vi "Digitizer Measurement.vi"(4 "delay (2.0 s)":dbl[unit]=2.0 format="%_3g", 6 "filepath":path, 7 "channel names":string="1,2", 8 "error in":errorcluster, 9 "trigger":T1={"trigger level"=30.0, "trigger type"=enum."Immediate", "Trigger Source"=enum."Immediate", "Trigger Slope"=enum."Positive"} {"trigger level" format="%.2f"}, 10 "vertical":T2={"vertical coupling"=enum."DC", "probe attenuation"=1.0, "vertical range"=10.0, "vertical offset"=0.0} {"vertical offset" format="%.4f"; "vertical range" format="%.2f"; "probe attenuation" format="%.1f"}, 11 "horizontal":T3={"number of records"=1, "reference position"=1.0, "min record length"=100000, "min sample rate"=1000000.0, "enforce realtime"=TRUE, "maximum input frequency"=-1.0} {"maximum input frequency" format="%.2f"; "min sample rate" step=1000000.0 format="%.0p"; "min record length" format="%.0p"; "reference position" format="%.1f"; "number of records" step=1}) -> (0 "error out":errorcluster, 2 "waveform array":waveform(dbl)[](array[waveform])=[{"t0"=timestamp(-9593225999.296875 s since 1904-01-01), "dt"=nan, "Y"=[]}, {"t0"=timestamp(3478177624.703125 s since 1904-01-01), "dt"=1e-06, "Y"=array[100000 elements]}])   [LabVIEW 2010]
doc: "This function performs Digitizer measurements (Configure, Read, and Close)."
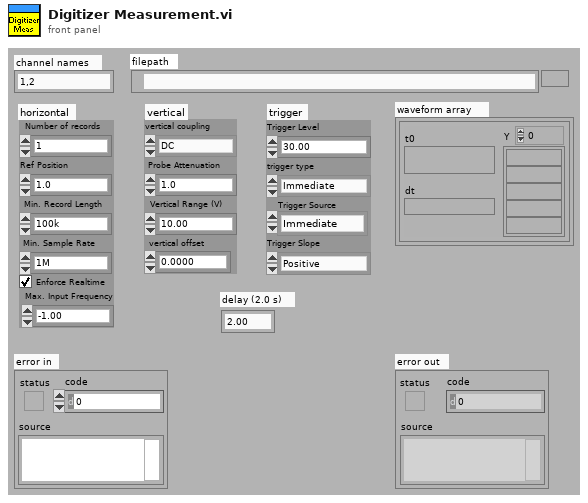
[diagram p1: front panel]
types:
  T1 = cluster{"trigger level":dbl, "trigger type":enum16{"Edge", "Digital", "Immediate"}, "Trigger Source":enum8{"Immediate", "Channel 0", "Channel 1", "Channel 2", "Channel 3", "Channel 4", "Channel 5", "Channel 6", "Channel 7", "External TRIG", "Software Trigger", "RTSI 0", "RTSI 1", "RTSI 2", "RTSI 3", "RTSI 4", "RTSI 5", "RTSI 6", "PFI 0", "PFI 1", "PFI 2", "PXI Star Trigger"}, "Trigger Slope":enum16{"Positive", "Negative"}}
  T2 = cluster{"vertical coupling":enum16{"AC", "DC", "Ground"}, "probe attenuation":dbl, "vertical range":dbl, "vertical offset":dbl}
  T3 = cluster{"number of records":i32, "reference position":dbl, "min record length":i32, "min sample rate":dbl, "enforce realtime":bool, "maximum input frequency":dbl}
  T4 = typedef "Typedef-Channel Parameters.ctl" = cluster{"Channel Name":string, "Number of Records":i32, "Reference Position":dbl, "Minimum Record Length":i32, "Minimum Sample Rate":dbl, "Maximum Input Frequency":dbl, "Enforce Realtime":bool, "Vertical Coupling":enum16{"AC", "DC", "Ground"}, "Probe Attenuation":dbl, "Vertical Range (V)":dbl, "Vertical Offset":dbl, "Trigger Level":dbl, "Trigger Type":enum16{"Edge", "Digital", "Immediate"}, "Trigger Source":enum16{"Immediate", "Channel 0", "Channel 1", "Channel 2", "Channel 3", "Channel 4", "Channel 5", "Channel 6", "Channel 7", "Extermal TRIG", "Software Trigger", "RTSI 0", "RTSI 1", "RTSI 2", "RTSI 3", "RTSI 4", "RTSI 5", "RTSI 6", "PF 0", "PF 1", "PF 2", "PXI Star Trigger"}, "Trigger Slope":enum16{"Positive", "Negative"}, "Digitizer 1 Used?":bool, "Digitizer 1 Channels":string, "Digitizer 1 Reference":refnum<k15>, "Digitizer 1 Gain Multiplier":dbl, "Digitizer 2 Used?":bool, "Digitizer 2 Channels":string, "Digitizer 2 Reference":refnum<k15>, "Session References":refnum<k20>[]}
  T5 = cluster{"relativeInitialX":dbl, "xIncrement":dbl, "wfm":dbl[]}[]
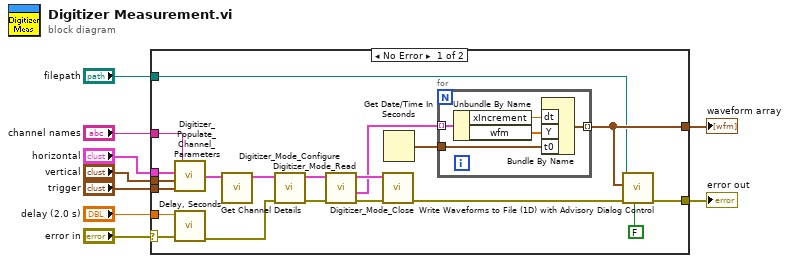
[diagram p0: block diagram]
diagram:
  n1 = case shown="No Error" "error in" {
    selector: "error in" -> [w12 w35]
    tunnel: "horizontal" -> [w29 _]
    tunnel: "vertical" -> [w28 _]
    tunnel: "trigger" -> [w27 _]
    tunnel: "channel names" -> [w26 _]
    tunnel: [w16 w35] -> w4
    tunnel: [w15 _] -> w3
    tunnel: "filepath" -> [w13 _]
    tunnel: "delay (2.0 s)" -> [w10 _]
    frame No Error {
      n2 = call "Digitizer_Populate_Channel_Parameters"("Trigger settings"=w27, "Vertical Settings"=w28, "Horizontal Settings"=w29, "Channel Name"=w26) -> ("Channel Parameters"=w25:T4)
      n3 = call "Delay, Seconds.vi"("error in"=w12, "delay"=w10) -> ("error out"=w11:errorcluster)  [unwired: 5 in, 1 out]
      n4 = call "Get Channel Details.vi"("Channel Parameters In"=w25) -> ("Channel Parameters Out"=w24:T4)  [unwired: 10 in]
      n5 = call "Digitizer_Mode_Configure.vi"("error in"=w11, "Channel Parameters In"=w24) -> ("error out"=w22:errorcluster, "Channel Parameters Out"=w21:T4)  [unwired: 7 in, 1 out]
      n6 = call "Digitizer_Mode_Read.vi"("error in"=w22, "Channel Parameters In"=w21) -> ("error out"=w23:errorcluster, "Waveforms Out"=w18:T5, "dup Channel Parameters Out"=w20:T4)  [unwired: 6 in, 1 out]
      n7 = call "Digitizer_Mode_Close.vi"("error in"=w23, "Channel Parameters In"=w20) -> ("error out"=w17:errorcluster)  [unwired: 7 in, 2 out]
      n8 = Get Date/Time In Seconds() -> (seconds since 1Jan1904=w19:timestamp)
      n9 = for {
        tunnel: w18 -> [w34] mode=indexing
        tunnel: [w31] -> w15 mode=indexing
        tunnel: w19 -> [w30]
        n10 = Unbundle By Name(w34) -> ("xIncrement"=w33:dbl, "wfm"=w32:dbl[])
        n11 = Bundle By Name("dt"=w33, "Y"=w32, "t0"=w30) -> (w31:waveform(dbl))  [unwired: 1 in]
      }
      n12 = call "Write Waveforms to File (1D) with Advisory Dialog Control.vi"("advisory dialog? (display:T)"=FALSE, "error in (no error)"=w17, "waveform array"=w15, "file path (dialog if empty)"=w13) -> ("error out"=w16:errorcluster)  [unwired: 6 in, 1 out]
    }
    frame Error {
    }
  }
  "error out" <- w4
  "waveform array" <- w3
